vi "Pump WP averaging test.vi"() -> ()   [LabVIEW 2013]
panel:
  out "At least N values?":bool
  out "Average (up to N)":dbl
  out "Array":dbl[](array[numeric])
  in  "N":i32
  out "0, 1":i16[](array[numeric])
  out "Number of values with specified photon #":i16
  in  "Photon #":dbl=300.0 format="%#_13g"
  in  "appended array":dbl[][](array[numeric])
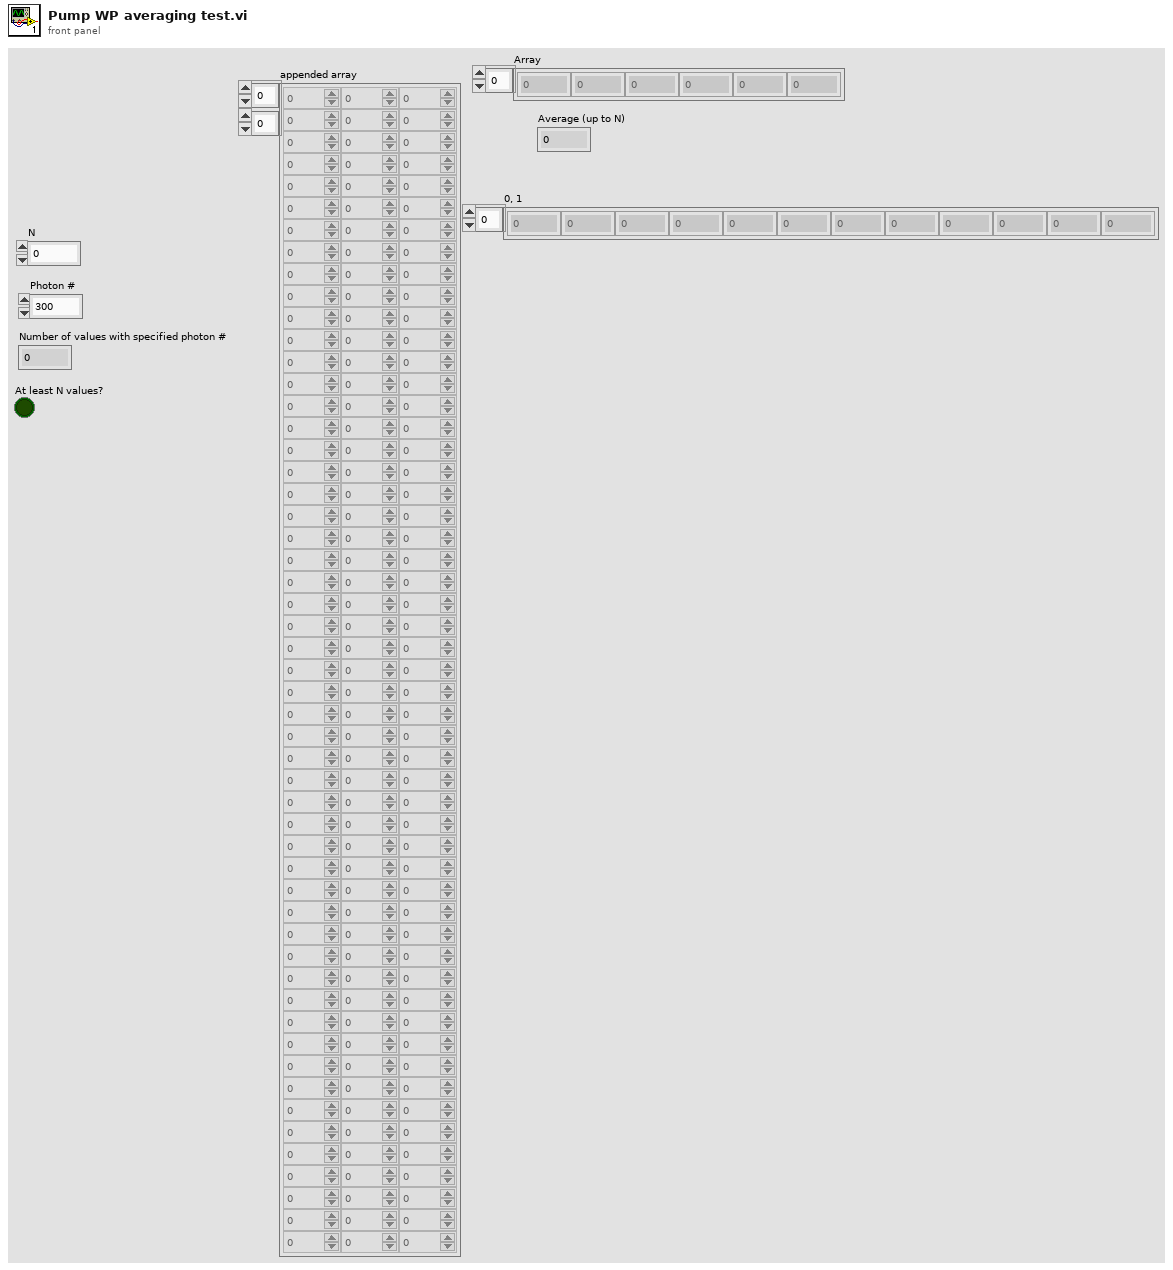
[diagram p1: front panel]
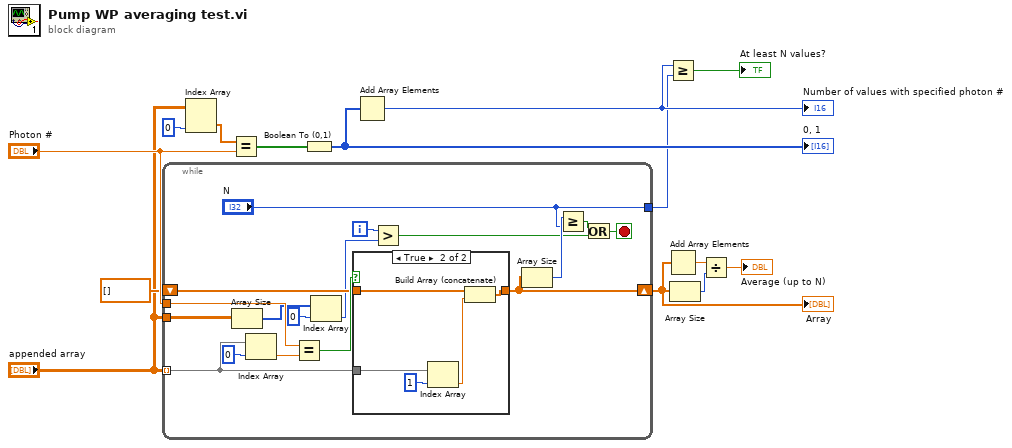
[diagram p0: block diagram]
diagram:
  n1 = while {
    tunnel: "appended array" -> [w27] mode=indexing
    tunnel: "Photon #" -> [w29]
    shift-right: [w25] -> w6
    shift-left: dbl[] [] -> [w26]
    tunnel: "appended array" -> [w23]
    tunnel: ["N"] -> w2
    i -> [w22]
    stop <- w16 stop-if-true
    n2 = Array Size(array=w23) -> (size(s)=w21:i32[])
    n3 = Index Array(array=w27, index=0) -> (element=w30:dbl)
    n4 = Equal?(x=w29, y=w30) -> (x = y?=w28:bool)
    n5 = Index Array(array=w21, index=0) -> (element=w19:i32)
    n6 = case shown="True" w28 {
      tunnel: w27 -> [_ w37]
      tunnel: [w32 w34] -> w25
      tunnel: w26 -> [w32 w33]
      frame False {
      }
      frame True {
        n7 = Index Array(array=w37, index=1) -> (element=w35:dbl)
        n8 = Build Array (concatenate)(w33, w35) -> (w34:dbl[])
      }
    }
    n9 = Greater?(x=w22, y=w19) -> (0:w18:bool)
    n10 = Array Size(array=w25) -> (size(s)=w24:i32)
    n11 = Greater Or Equal?(x=w24, y="N") -> (x >= y?=w17:bool)
    n12 = Or(x=w17, y=w18) -> (x .or. y?=w16:bool)
  }
  "Array" <- w6
  n13 = Index Array(array="appended array", index (col)=0 ("disabled index (col)")) -> (element=w11:dbl[])  [unwired: 1 in]
  n14 = Equal?(x=w11, y="Photon #") -> (x = y?=w14:bool[])
  n15 = Boolean To (0,1)(Boolean=w14) -> (0, 1=w13:i16[])
  "0, 1" <- w13
  n16 = Add Array Elements(numeric array=w13) -> (sum=w3:i16)
  "Number of values with specified photon #" <- w3
  n17 = Greater Or Equal?(x=w3, y=w2) -> (x >= y?=→"At least N values?":bool)
  n18 = Add Array Elements(numeric array=w6) -> (sum=w7:dbl)
  n19 = Array Size(array=w6) -> (size(s)=w5:i32)
  n20 = Divide(x=w7, y=w5) -> (x/y=→"Average (up to N)":dbl)
